vi "TrafficObstacles.vi"(8 "error in":errorcluster) -> (0 "error out":errorcluster, 1 "Obstacle":bool, 2 "Green Light":bool, 3 "Red Light":bool, 4 "Unprocessed Webcam Feed":T1(plugin-control), 5 "Processed Traffic Light":T1(plugin-control), 6 "Obstacle Circles Data":T4(array[cluster]), 7 "Processed Obstacles":T1(plugin-control))   [LabVIEW 2015]
uses:
  HueSlider.ctl
  <vilib>/vision/NI_Vision_Development_Module.lvlib
panel:
  in  "?":enum32{"Detection Settings", "Camera Settings"}(tab)
  in  "Obstacle Hue range":T2={"Min"=1, "Max"=11} scale=0.0..255.0
  in  "Traffic Light Brightness":cluster{"Lower value":sgl, "Upper value":sgl}={"Lower value"=235.0, "Upper value"=255.0}
  in  "Traffic Light Min Radius":sgl=9.0
  in  "Traffic Light Max Radius":sgl=20.0
  in  "Obstacle Min Radius":sgl=9.0
  in  "Obstacle Max Radius":sgl=29.0
  in  "Exposure::Value":i64=600 min=1 max=5000 step=1
  in  "White Balance::Value":i64=3200 min=2800 max=6500 step=1
  in  "White Balance::Mode":u32(ring) items=["Manual", "Auto"]
  in  "?":enum32{" Results", "Detailed Data"}(tab)
  out "Process Time":dbl
  out "Red Histogram Report - Obstacle":T3 {"Standard  Variation" format="%.2f"; "Mean Value" format="%.2f"; "Interval Width" format="%.2f"; "Starting Value" format="%.2f"; "Maximal Value" format="%.2f"; "Minimal Value" format="%.2f"}
  out "Blue  Histogram Report - Obstacle":T3 {"Standard  Variation" format="%.2f"; "Mean Value" format="%.2f"; "Interval Width" format="%.2f"; "Starting Value" format="%.2f"; "Maximal Value" format="%.2f"; "Minimal Value" format="%.2f"}
  out "Traffic Signal Circles Data":T4(array[cluster])
  out "Red Histogram Report - Traffic Signal":T3 {"Standard  Variation" format="%.2f"; "Mean Value" format="%.2f"; "Interval Width" format="%.2f"; "Starting Value" format="%.2f"; "Maximal Value" format="%.2f"; "Minimal Value" format="%.2f"}
  out "Blue  Histogram Report - Traffic Signal":T3 {"Standard  Variation" format="%.2f"; "Mean Value" format="%.2f"; "Interval Width" format="%.2f"; "Starting Value" format="%.2f"; "Maximal Value" format="%.2f"; "Minimal Value" format="%.2f"}
  out "Circle Count - Obstacle":i32
  out "Circle Count - Traffic Signal":i32
  # "Recommended Settings: \n\nTraffic Light Brightness: 240 (or higher) - 255 depending on the exposure value you may increase the lower bound\n\nTraffic Light Radius: 9 - 15\n\nObstacel Hue Range: 1- 10 (caliberate this range based on the given enviroment) \n\nObstacke Radius: 10 - 18"
  # "Recommended Settings: \n\nExposure: 650 - 750\nWhite Balance: 4400 - 5000\nWhite Balance Mode: Manual\nCamera Resolution: 176 X 144 (set inside the Vision Aquisition block)"
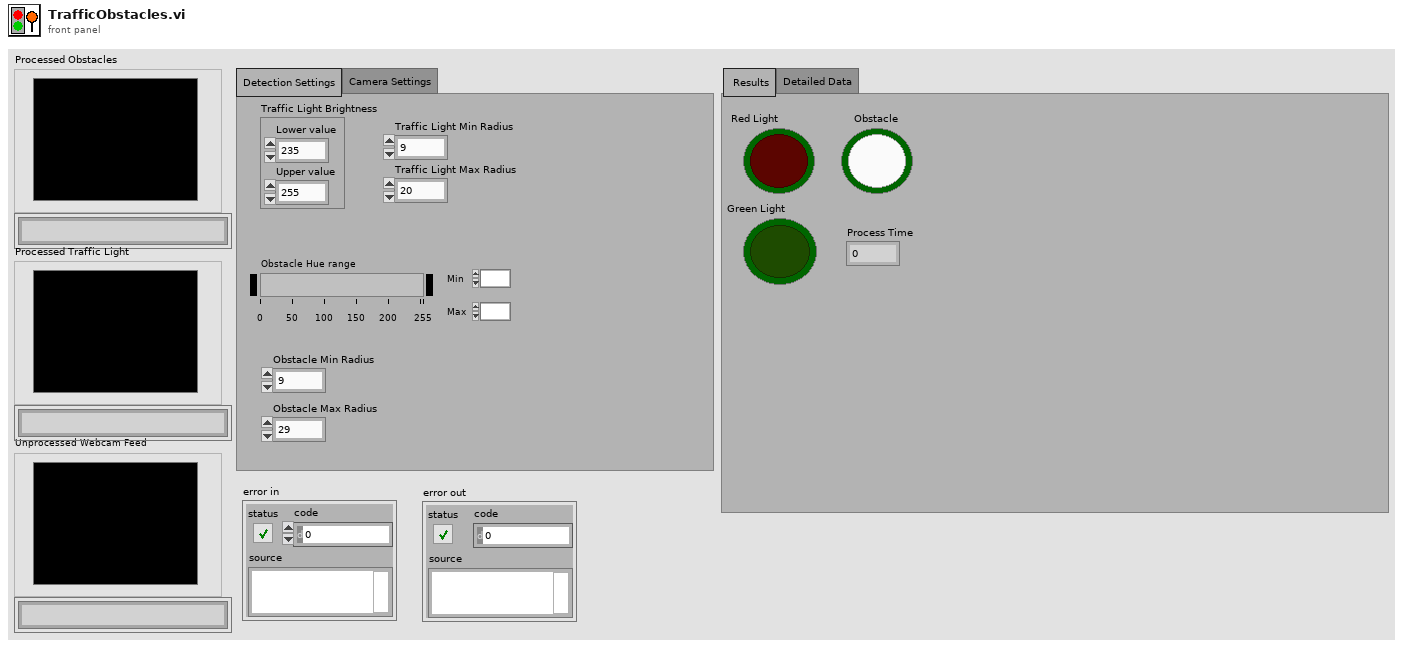
[diagram p1: front panel]
types:
  T1 = typedef "IMAQ Image.ctl" = refnum<image>
  T2 = typedef "HueSlider.ctl" = cluster{"Min":i32, "Max":i32}
  T3 = cluster{"histogram":u32[], "Minimal Value":sgl, "Maximal Value":sgl, "Starting Value":sgl, "Interval Width":sgl, "Mean Value":sgl, "Standard  Variation":sgl, "Area (pixels)":i32}
  T4 = cluster{"Pos. X":i32, "Pos. Y":i32, "Radius":i32, "Core Area":i32}[]
  T5 = typedef "IMAQ Circle" = cluster{"Center X":i32, "Center Y":i32, "Inner Radius":i32, "Outer Radius":i32, "Start Angle":dbl, "End Angle":dbl}
  T6 = cluster{"Pos. X":i32, "Pos. Y":i32, "Radius":i32, "Core Area":i32}
  T7 = typedef "ROI Descriptor" = cluster{"Global Rectangle":i32[], "Contours":cluster{"ID":enum32{"External", "Internal"}, "Type":u32, "Coordinates":i32[]}[]}
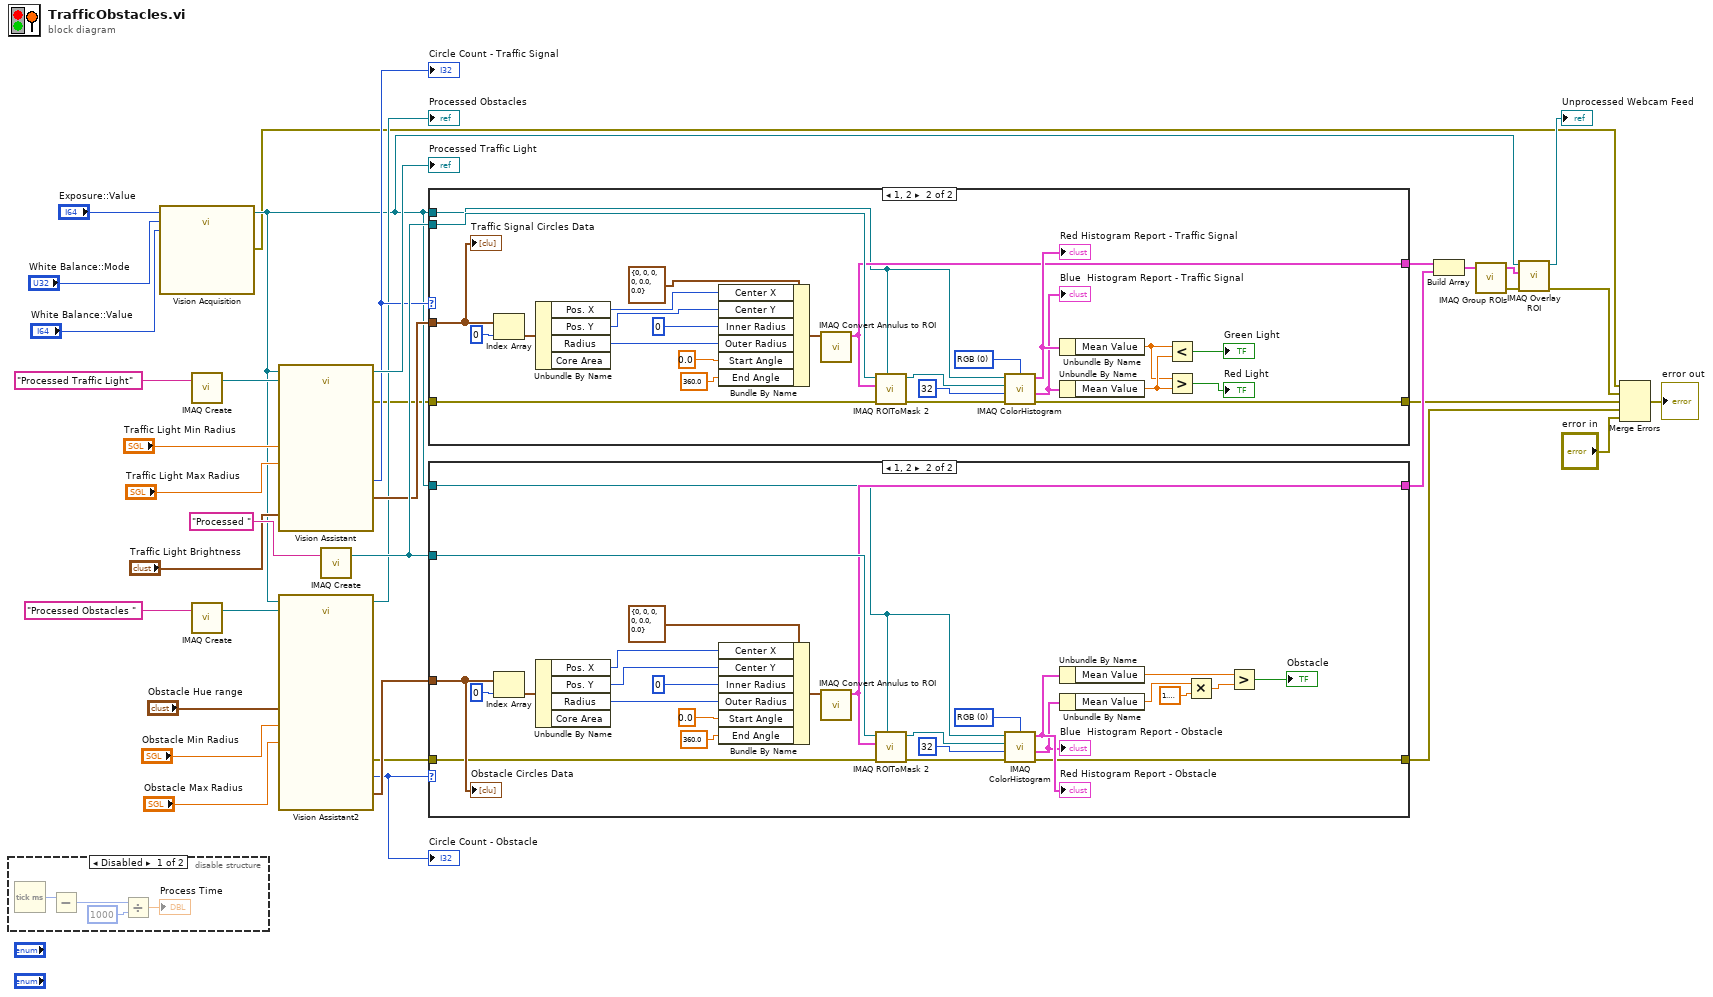
[diagram p0: block diagram]
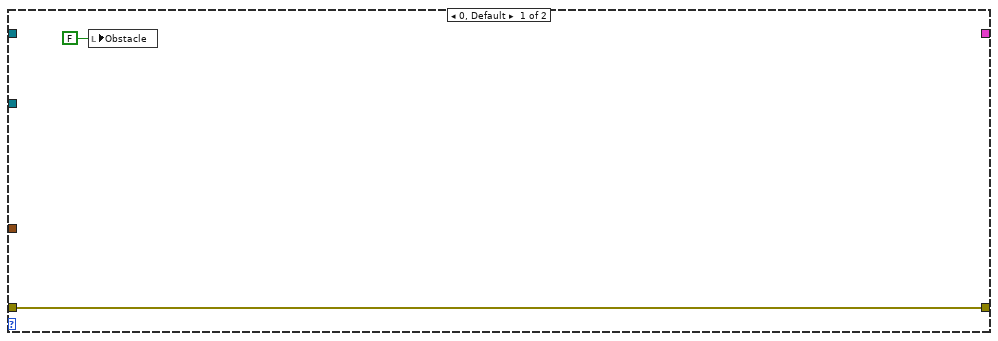
[diagram p3: hidden frame]
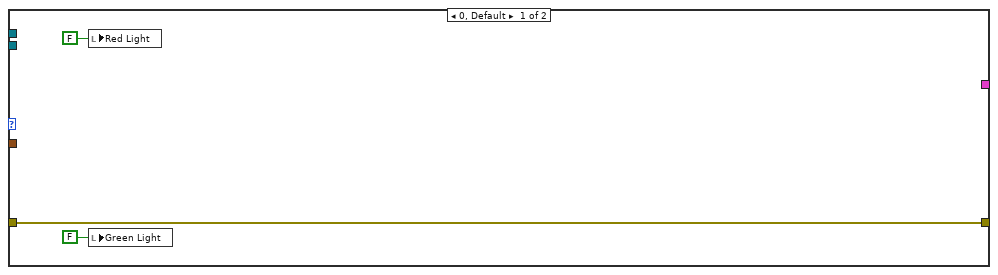
[diagram p4: hidden frame]
diagram:
  n1 = disable-structure shown="Disabled" {
    frame Disabled {
      n2 = Tick Count (ms)() -> (millisecond timer value=w37:u32)
      n3 = Subtract(x=w37) -> (x-y=w40:u32)  [unwired: 1 in]
      n4 = Divide(x=w40, y=u32 1000) -> (x/y=→"Process Time":dbl)
    }
    frame Enabled {
    }
  }
  n5 = call "Vision Acquisition"("Exposure::Value"="Exposure::Value", "White Balance::Mode"="White Balance::Mode", "White Balance::Value"="White Balance::Value") -> ("Image Out"=w12:T1, "error out"=w1:errorcluster)  [unwired: 22 in, 1 out]
  n6 = call "IMAQ Create"("Image Name"="Processed Traffic Light") -> ("New Image"=w35:T1)  [unwired: 3 in, 2 out]
  n7 = call "IMAQ Create"("Image Name"="Processed Obstacles ") -> ("New Image"=w31:T1)  [unwired: 3 in, 2 out]
  n8 = call "Vision Assistant"("Image In"=w12, "Image Dst"=w35, "Min Radius (Circle Detection 1)"="Traffic Light Min Radius", "Max Radius (Circle Detection 1)"="Traffic Light Max Radius", "Range (Threshold 1)"="Traffic Light Brightness") -> ("Image Out"=→"Processed Traffic Light":T1, "Circles Data (Circle Detection 1)"=w28:T4, "error out"=w6:errorcluster, "Nb Circles (Circle Detection 1)"=w26:i32)  [unwired: 3 in, 16 out]
  "Circle Count - Traffic Signal" <- w26
  n9 = call "Vision Assistant2"("Image In"=w12, "Image Dst"=w31, "Range (Threshold 1)"="Obstacle Hue range", "Min Radius (Circle Detection 1)"="Obstacle Min Radius", "Max Radius (Circle Detection 1)"="Obstacle Max Radius") -> ("Image Out"=→"Processed Obstacles":T1, "Nb Circles (Circle Detection 1)"=w18:i32, "Circles Data (Circle Detection 1)"=w19:T4, "error out"=w7:errorcluster)  [unwired: 19 in]
  "Circle Count - Obstacle" <- w18
  n10 = call "IMAQ Create"("Image Name"="Processed ") -> ("New Image"=w33:T1)  [unwired: 3 in, 2 out]
  n11 = case shown="1, 2" w26 {
    tunnel: w28 -> [_ w69]
    tunnel: w33 -> [_ w55]
    tunnel: [_ w48] -> w14
    tunnel: w12 -> [_ w47]
    tunnel: w6 -> [w43 w46]
    tunnel: [w43 w44] -> w3
    frame 0, Default {
      n12 = local write "Red Light"(FALSE ("Traffic Light - Red")) -> ()
      n13 = local write "Green Light"(FALSE ("Traffic Light - Green")) -> ()
    }
    frame 1, 2 {
      w57 = u16 0 items=["RGB", "HSL", "HSV", "HSI", "CIE L*a*b*", "CIE XYZ"] ("Color Mode")
      n14 = Index Array(array=w69, index=0) -> (element=w65:T6)
      n15 = Unbundle By Name(w65) -> ("Pos. X"=w67:i32, "Pos. Y"=w66:i32, "Radius"=w63:i32)  [unwired: 1 out]
      n16 = Bundle By Name(cluster=T5 {"Center X"=0, "Center Y"=0, "Inner Radius"=0, "Outer Radius"=0, "Start Angle"=0.0, "End Angle"=0.0} ("Annulus"), "Center X"=w67, "Center Y"=w66, "Inner Radius"=0, "Outer Radius"=w63, "Start Angle"=0.0, "End Angle"=360.0) -> (w59:T5)
      n17 = call "IMAQ Convert Annulus to ROI"("Annulus"=w59) -> ("ROI Descriptor"=w48:T7)  [unwired: 8 in, 1 out]
      n18 = call "IMAQ ROIToMask 2"("Image Model"=w47, "error in (no error)"=w46, "ROI Descriptor"=w48, "Image"=w55) -> ("error out"=w45:errorcluster, "Image Out"=w58:T1)  [unwired: 5 in, 1 out]
      n19 = call "IMAQ ColorHistogram"("Color Mode"=w57, "Image Src"=w47, "Image Mask"=w58, "Number of Classes"=32, "error in (no error)"=w45) -> ("Red or Hue or X or L* Histogram Report"=w54:T3, "Blue or Luma or Val or Inten or Z or b* Histogram Report"=w49:T3, "error out"=w44:errorcluster)  [unwired: 1 in, 1 out]
      "Red Histogram Report - Traffic Signal" <- w54
      "Blue  Histogram Report - Traffic Signal" <- w49
      n20 = Unbundle By Name(w54) -> ("Mean Value"=w51:sgl)
      n21 = Unbundle By Name(w49) -> ("Mean Value"=w52:sgl)
      n22 = Less?(x=w51, y=w52) -> (x < y?=→"Green Light":bool)
      n23 = Greater?(x=w51, y=w52) -> (0:→"Red Light":bool)
      "Traffic Signal Circles Data" <- w69
    }
  }
  n24 = case shown="1, 2" w18 {
    tunnel: w19 -> [_ w98]
    tunnel: w33 -> [_ w84]
    tunnel: w12 -> [_ w80]
    tunnel: [_ w81] -> w15
    tunnel: w7 -> [w71 w73]
    tunnel: [w71 w72] -> w4
    frame 0, Default {
      n25 = local write "Obstacle"(FALSE ("Obstacle")) -> ()
    }
    frame 1, 2 {
      w86 = u16 0 items=["RGB", "HSL", "HSV", "HSI", "CIE L*a*b*", "CIE XYZ"] ("Color Mode")
      n26 = Index Array(array=w98, index=0) -> (element=w94:T6)
      n27 = Unbundle By Name(w94) -> ("Pos. X"=w96:i32, "Pos. Y"=w95:i32, "Radius"=w92:i32)  [unwired: 1 out]
      n28 = Bundle By Name(cluster=T5 {"Center X"=0, "Center Y"=0, "Inner Radius"=0, "Outer Radius"=0, "Start Angle"=0.0, "End Angle"=0.0} ("Annulus"), "Center X"=w96, "Center Y"=w95, "Inner Radius"=0, "Outer Radius"=w92, "Start Angle"=0.0, "End Angle"=360.0) -> (w88:T5)
      n29 = call "IMAQ Convert Annulus to ROI"("Annulus"=w88) -> ("ROI Descriptor"=w81:T7)  [unwired: 8 in, 1 out]
      n30 = call "IMAQ ROIToMask 2"("Image Model"=w80, "error in (no error)"=w73, "ROI Descriptor"=w81, "Image"=w84) -> ("error out"=w74:errorcluster, "Image Out"=w87:T1)  [unwired: 5 in, 1 out]
      n31 = call "IMAQ ColorHistogram"("Color Mode"=w86, "Image Src"=w80, "Image Mask"=w87, "Number of Classes"=32, "error in (no error)"=w74) -> ("Red or Hue or X or L* Histogram Report"=w83:T3, "Blue or Luma or Val or Inten or Z or b* Histogram Report"=w82:T3, "error out"=w72:errorcluster)  [unwired: 1 in, 1 out]
      "Red Histogram Report - Obstacle" <- w83
      "Blue  Histogram Report - Obstacle" <- w82
      n32 = Unbundle By Name(w83) -> ("Mean Value"=w77:sgl)
      n33 = Unbundle By Name(w82) -> ("Mean Value"=w79:sgl)
      n34 = Multiply(x=w79, y=sgl 1.9) -> (x*y=w76:sgl)
      n35 = Greater?(x=w77, y=w76) -> (0:→"Obstacle":bool)
      "Obstacle Circles Data" <- w98
    }
  }
  n36 = Build Array(w14, w15) -> (w13:T7[])
  n37 = call "IMAQ Group ROIs"("ROI Descriptors"=w13) -> ("error out"=w5:errorcluster, "ROI Descriptor out"=w16:T7)  [unwired: 3 in]
  n38 = call "IMAQ Overlay ROI"("error in (no error)"=w5, "ROI Descriptor"=w16, "Image"=w12) -> ("error out"=w2:errorcluster, "Image Out"=→"Unprocessed Webcam Feed":T1)  [unwired: 7 in]
  n39 = Merge Errors(w1, w2, w3, w4, "error in") -> (→"error out":errorcluster)
